vi "Get Array Values as Strings.vi"(8 "error in (no error)":errorcluster, 11 "JSON Value in":refnum<class "JSON Value.lvclass">) -> (0 "error out":errorcluster, 3 "values":string[](array[string]))   [LabVIEW 2016, in "JSON Value.lvclass"]
doc: "Returns the element type of each element in a JSON Array. If all elements are of the same type, single type is true."
uses:
  JSON Value.lvclass
  JSON Types.ctl
  subVIs/Errors.ctl
  Read Value/Read value as String.vi
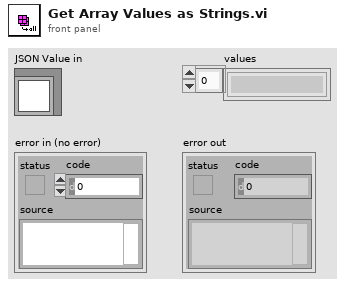
[diagram p1: front panel]
types:
  T1 = typedef "JSON Value.lvclass/JSON Types.ctl" = enum16{"String", "Numeric", "Boolean", "NULL", "Object", "Array"}
  T2 = typedef "JSON Value.lvclass/Errors.ctl" = enum16{"No key", "Key path type", "Array OOB", "Type Mismatch", "Invalid Token"}
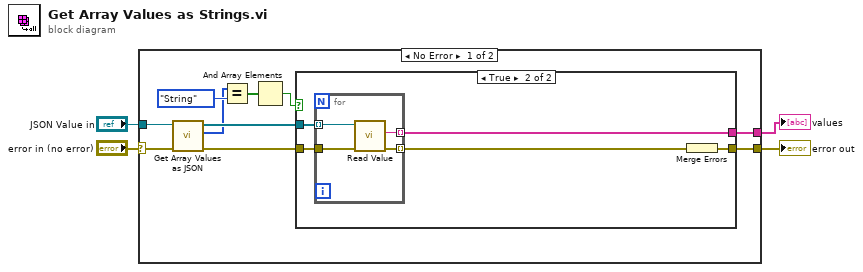
[diagram p0: block diagram]
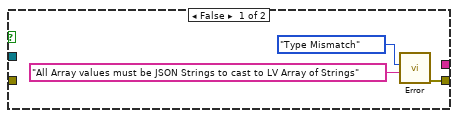
[diagram p2: hidden frame]
diagram:
  n1 = case shown="No Error" "error in (no error)" {
    selector: "error in (no error)" -> [w13 w27]
    tunnel: "JSON Value in" -> [w14 _]
    tunnel: [w11 w27] -> w2
    tunnel: [w9 _] -> w1
    frame No Error {
      n2 = call "Get Array Values as JSON.vi"("error in (no error)"=w13, "JSON Value in"=w14) -> ("error out"=w8:errorcluster, "types"=w7:T1[], "values"=w12:refnum<class "JSON Value.lvclass">[])  [unwired: 6 in, 1 out]
      n3 = Equal?(x=w7, y=JSON_Types."String") -> (x = y?=w6:bool[])
      n4 = And Array Elements(Boolean array=w6) -> (logical AND=w5:bool)
      n5 = case shown="True" w5 {
        tunnel: w12 -> [_ w22]
        tunnel: [w15 w18] -> w11
        tunnel: [_ w21] -> w9
        tunnel: w8 -> [_ w19]
        frame False {
          n6 = call "Error.vi"("Data"="All Array values must be JSON Strings to cast to LV Array of Strings", 9:Errors."Type Mismatch") -> ("error out"=w15:errorcluster)  [unwired: 8 in]
        }
        frame True {
          n7 = for {
            tunnel: w22 -> [w23] mode=indexing
            tunnel: [w26] -> w21 mode=indexing
            tunnel: [w25] -> w20 mode=indexing
            tunnel: w19 -> [w24]
            n8 = call-poly "Read Value.vi"("error in (no error)"=w24, "JSON String in"=w23) -> ("error out"=w25:errorcluster, "value"=w26:string)  [unwired: 8 in]
          }
          n9 = Merge Errors(w20) -> (w18:errorcluster)
        }
      }
    }
    frame Error {
    }
  }
  "error out" <- w2
  "values" <- w1
